vi "Write Default Timeout (ms).vi"(8 "error in (no error)":errorcluster, 10 "Default Timeout (ms)":i32=-1, 11 "Event_Bus in":refnum<class "Event_Bus.lvclass">) -> (0 "error out":errorcluster, 3 "Event_Bus out":refnum<class "Event_Bus.lvclass">)   [LabVIEW 2021, in "Event_Bus.lvclass"]
uses:
  Event_Bus.lvclass
  Event_Bus.lvclass/Event_Bus.ctl
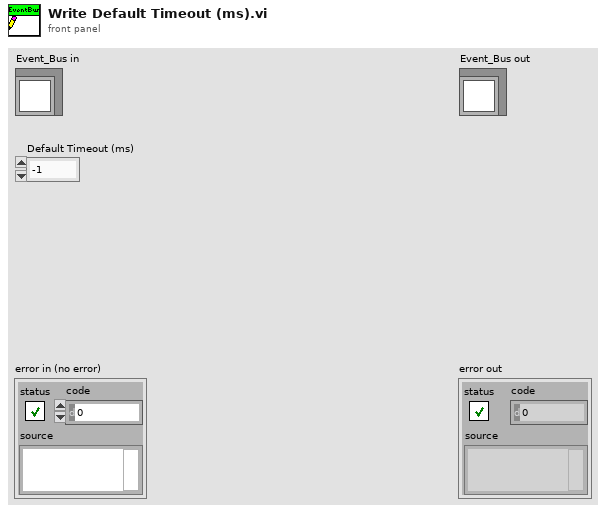
[diagram p1: front panel]
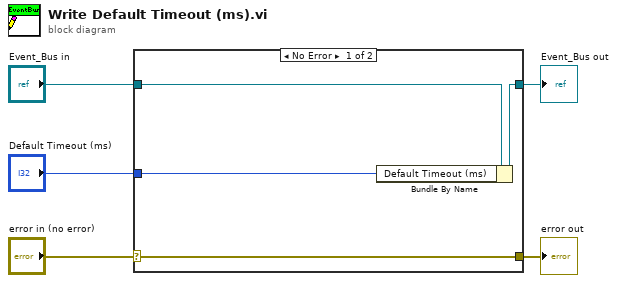
[diagram p0: block diagram]
diagram:
  n1 = case shown="No Error" "error in (no error)" {
    selector: "error in (no error)" -> [w9 w10]
    tunnel: [w9 w10] -> w4
    tunnel: [w7 w11] -> w2
    tunnel: "Event_Bus in" -> [w8 w11]
    tunnel: "Default Timeout (ms)" -> [w6 _]
    frame No Error {
      n2 = Bundle By Name(cluster=w8, "Default Timeout (ms)"=w6) -> (w7:refnum<class "Event_Bus.lvclass">)
    }
    frame Error {
    }
  }
  "error out" <- w4
  "Event_Bus out" <- w2
